vi "RSZVB Set Coherent Signal Phase.vi"(7 "Phase (0.0 deg)":dbl format="%^.3e", 8 "error in (no error)":errorcluster {"code" format="%.0x"}, 9 "Port (1)":i32=1, 10 "Channel (1)":i32=1, 11 "VISA session":refnum<visa-resource-name>) -> (0 "error out":errorcluster {"code" format="%.0x"}, 3 "dup VISA session":refnum<visa-resource-name>)   [LabVIEW 2011]
doc: "This VI defines the phase for the coherent signal at port no. <Pt> relative to the phase of the reference signal (SOURce<Ch>:CMODe:RPORt). \n\nNote(s):\n\n(1) This VI is not available for R&S ZVB instrument.\n\nRemote-control command(s):\nSOURce<Ch>:CMODe:PORT<Pt>:PHASe"
uses:
  _utility/RSZVB Global Data.vi
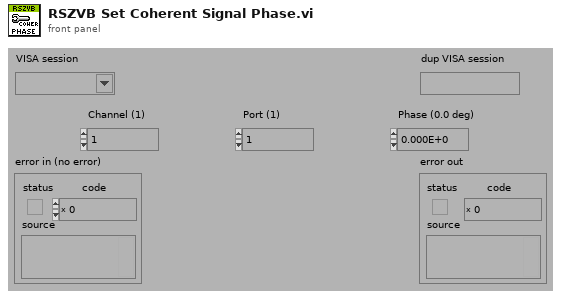
[diagram p1: front panel]
types:
  T1 = cluster{"Error Checking (T: On)":bool, "Installed Options":string[], "Data Valid?":bool, "Ports":i32, "Model":string[], "Option Checking (T: On)":bool}[]
  T2 = cluster{"Error Checking (T: On)":bool, "Installed Options":string[], "Data Valid?":bool, "Ports":i32, "Model":string[], "Option Checking (T: On)":bool}
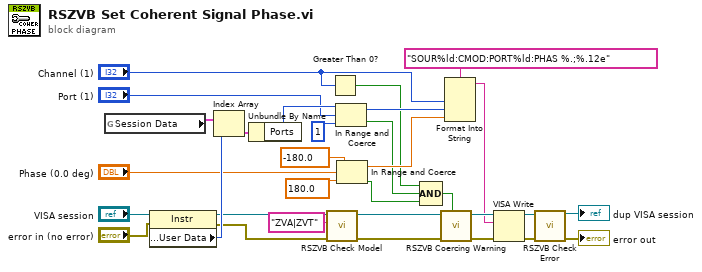
[diagram p0: block diagram]
diagram:
  n1 = global read "RSZVB Global Data.vi" "Session Data"() -> (w22:T1)
  n2 = property class="Instr"(reference="VISA session", error in="error in (no error)") -> (reference out=w2:refnum<visa-resource-name>, error out=w1:errorcluster, "General Settings:User Data"=w24:u32)
  n3 = Index Array(array=w22, index=w24) -> (element=w21:T2)
  n4 = Unbundle By Name(w21) -> ("Ports"=w25:i32)
  n5 = call "RSZVB Check Model.vi"("error in (no error)"=w1, "Model"="ZVA|ZVT", "VISA session"=w2) -> ("error out"=w3:errorcluster, "dup VISA session"=w4:refnum<visa-resource-name>)  [unwired: 7 in]
  n6 = Greater Than 0?(x="Channel (1)") -> (x > 0?=w13:bool)
  n7 = In Range and Coerce(upper limit=w25, x="Port (1)", lower limit=1) -> (coerced(x)=w26:i32, In Range?=w14:bool)
  n8 = In Range and Coerce(upper limit=-180.0 ("lower limit"), x="Phase (0.0 deg)", lower limit=180.0) -> (coerced(x)=w30:dbl, In Range?=w31:bool)
  n9 = Compound Arithmetic op=AND(w13, w14, w31) -> (w27:bool)
  n10 = call "RSZVB Coercing Warning.vi"("In Range?"=w27, "error in (no error)"=w3, "VISA session"=w4) -> ("error out"=w18:errorcluster, "dup VISA session"=w19:refnum<visa-resource-name>)  [unwired: 7 in]
  n11 = Format Into String(format string="SOUR%ld:CMOD:PORT%ld:PHAS %.;%.12e", "Channel (1)", w26, w30) -> (resulting string=w17:string)  [unwired: 2 in, 1 out]
  n12 = VISA Write(VISA resource name=w19, write buffer=w17, error in (no error)=w18) -> (VISA resource name out=w16:refnum<visa-resource-name>, error out=w15:errorcluster)  [unwired: 1 out]
  n13 = call "RSZVB Check Error.vi"("error in (no error)"=w15, "VISA session"=w16) -> ("error out"=→"error out":errorcluster, "dup VISA session"=→"dup VISA session":refnum<visa-resource-name>)  [unwired: 8 in]
